vi "Prepare Control.vi"(7 "VolatusAPI":refnum<class "VolatusAPI.lvclass">, 8 "error in (no error)":errorcluster, 11 "LatchedValve in":refnum<class "LatchedValve.lvclass">) -> (0 "error out":errorcluster, 3 "LatchedValve out":refnum<class "LatchedValve.lvclass">)   [LabVIEW 2020, in "VolatusControl.lvlib" / "LatchedValve.lvclass"]
uses:
  LatchedValve.lvclass
  Volatus/VolatusAPI/VolatusAPI.lvclass
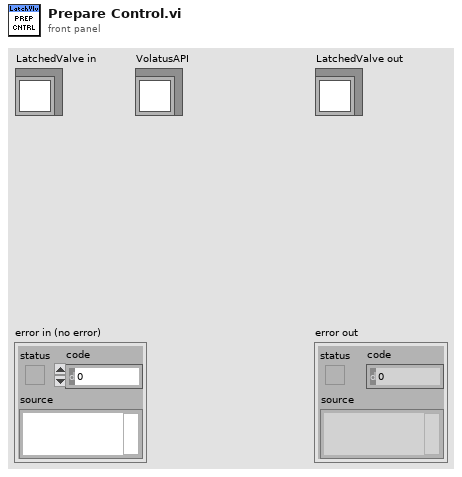
[diagram p1: front panel]
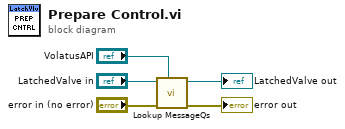
[diagram p0: block diagram]
diagram:
  n1 = call "Lookup MessageQs.vi"("VolatusAPI"="VolatusAPI", "error in (no error)"="error in (no error)", "LatchedValve in"="LatchedValve in") -> ("error out"=→"error out":errorcluster, "LatchedValve out"=→"LatchedValve out":refnum<class "LatchedValve.lvclass">)  [unwired: 7 in]
